vi "Str2Num.vi"(10 "Array in":string[](array[string]), 11 "Array 3":i32[](array[numeric])) -> (3 "Array out":i32[](array[numeric]))   [LabVIEW 2015]
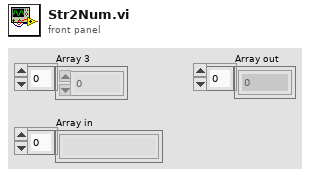
[diagram p1: front panel]
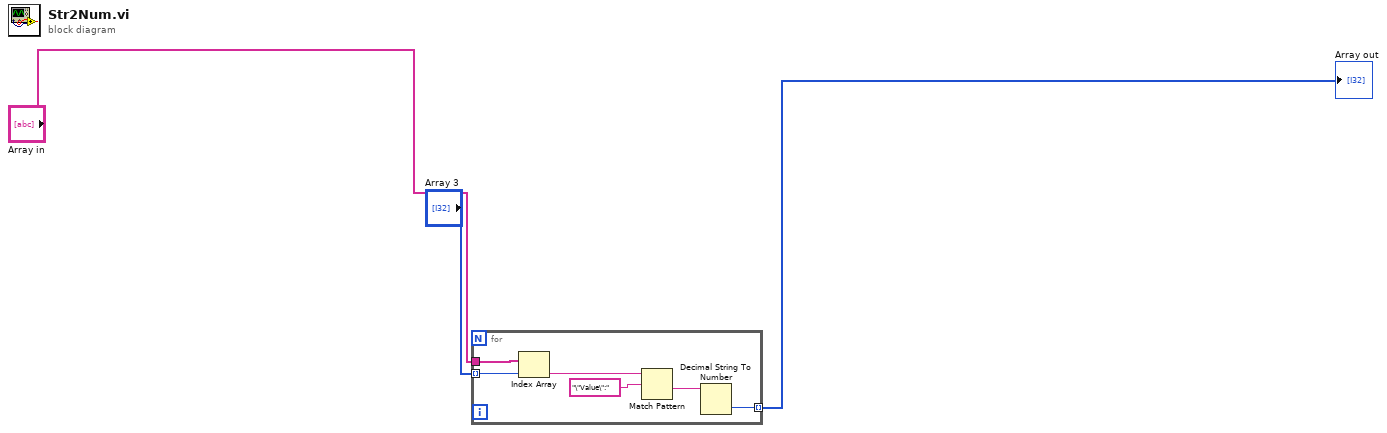
[diagram p0: block diagram]
diagram:
  n1 = for {
    tunnel: "Array 3" -> [w9] mode=indexing
    tunnel: [w6] -> w2 mode=indexing
    tunnel: "Array in" -> [w5]
    n2 = Index Array(array=w5, index=w9) -> (element=w4:string)
    n3 = Match Pattern(string=w4, regular expression="\"Value\":") -> (after substring=w7:string)  [unwired: 1 in, 3 out]
    n4 = Decimal String To Number(string=w7) -> (number=w6:i32)  [unwired: 2 in, 1 out]
  }
  "Array out" <- w2
